vi "S4GUI_003.vi"(7 "Tab ObsEng":enum32{"Obs", "CCD modes", "Guider", "Eng"}(tab)) -> ()   [LabVIEW 2018] (continued)
                w2587 = enum16{"OFF", "ON"}."OFF" ("Frame Transfer")
                n1481 = property on="Frame Transfer" class="Enum (strict)"(error in=w2589, "DisabledEnum"=T12."Disabled and Grayed Out" ("Disabled"), "Value"=w2587) -> (error out=w2588:errorcluster)  [unwired: 1 in, 1 out]
              }
            }
            n1482 = property on="FT warning" class="Str"("Caption.Visible"=w2543) -> ()  [unwired: 2 in, 2 out]
            n1483 = call-dynamic "Write mode Adm.vi"("error in (no error)"=w2550, "mode Adm"=FALSE, "S4GUI in"=w2546) -> ("error out"=w2576:errorcluster, "S4GUI out"=w2578:refnum<class "S4GUI.lvclass">)  [unwired: 7 in]
            n1484 = local write "password 2"("" ("password")) -> ()
            n1485 = call-dynamic "Write SET request.vi"("error in (no error)"=w2576, "SET request"=FALSE, "S4GUI in"=w2578) -> ("error out"=w2575:errorcluster, "S4GUI out"=w2577:refnum<class "S4GUI.lvclass">)  [unwired: 7 in]
            n1486 = disable-structure shown="Disabled" {
              frame Disabled {
                n1487 = flat-sequence {
                  tunnel: _ -> [w2597]
                  tunnel: [w2597] -> _
                  frame #0 {
                    n1488 = local read "AQM"() -> (w2594:T4)
                    n1489 = Less Or Equal?(x=w2594, y=T4."NORMAL FAINT: Conventional; 1 MHz; Gain 2") -> (x <= y?=w2593:bool)
                    n1490 = Select(t=w2594, s=w2593, f=T4."SLOW BRIGHT: Conventional; 0.1 MHz; Gain 1" ("y")) -> (s? t:f=w2595:T4)
                    n1491 = local write "EM Gain"(u16 2 ("EM Gain")) -> ()
                    n1492 = local write "AQM"(w2595) -> ()
                  }
                }
              }
              frame Enabled {
              }
            }
            n1493 = flat-sequence {
              tunnel: w2575 -> [w2600]
              tunnel: [w2600] -> w2561
              tunnel: [w2599] -> w2558
              tunnel: [w2598] -> w2559
              frame #0 {
                w2598 = u16 2 ("EM Gain")
                w2599 = T4."NORMAL FAINT: Conventional; 1 MHz; Gain 2" ("AQM")
                n1494 = local write "EM Gain"(w2598) -> ()
                n1495 = local write "AQM"(w2599) -> ()
              }
            }
            n1496 = call-dynamic "Read CCD mode.vi"("error in (no error)"=w2561, "S4GUI in"=w2577) -> ("error out"=w2566:errorcluster, "CCD mode"=w2564:T30, "S4GUI out"=w2563:refnum<class "S4GUI.lvclass">)  [unwired: 7 in]
            n1497 = local read "SZM"() -> (w2560:T3)
            n1498 = Bundle By Name(cluster=w2564, "FTM"=w2544, "SZM"=w2560, "EM gain"=w2559, "AQM"=w2558) -> (w2565:T30)
            n1499 = call-dynamic "Write CCD mode.vi"("error in (no error)"=w2566, "CCD mode"=w2565, "S4GUI in"=w2563) -> ("error out"=w2568:errorcluster, "S4GUI out"=w2567:refnum<class "S4GUI.lvclass">)  [unwired: 7 in]
            n1500 = call-dynamic "LoadCCDmode.vi"("error in (no error)"=w2568, "S4GUI in"=w2567) -> ("error out"=w2570:errorcluster, "S4GUI out"=w2569:refnum<class "S4GUI.lvclass">)  [unwired: 8 in]
            n1501 = call-dynamic "Read Parameters CCD modes.vi"("error in (no error)"=w2570, "S4GUI in"=w2569) -> ("error out"=w2573:errorcluster, "Parameters CCD modes"=w2562:T5, "S4GUI out"=w2571:refnum<class "S4GUI.lvclass">)  [unwired: 7 in]
            n1502 = local write "Parameters CCD modes"(w2562) -> ()
            n1503 = call-dynamic "Read InfoCCDmode.vi"("error in (no error)"=w2573, "S4GUI in"=w2571) -> ("error out"=w2556:errorcluster, "InfoCCDmode"=w2572:T2, "S4GUI out"=w2557:refnum<class "S4GUI.lvclass">)  [unwired: 7 in]
            n1504 = local write "InfoCCDmode"(w2572) -> ()
            n1505 = call-dynamic "CalcTemp.vi"("error in (no error)"=w2556, "S4GUI in"=w2557) -> ("error out"=w2555:errorcluster, "S4GUI out"=w2553:refnum<class "S4GUI.lvclass">)  [unwired: 8 in]
            n1506 = call-dynamic "Read Prev Temp.vi"("error in (no error)"=w2555, "S4GUI in"=w2553) -> ("error out"=w2554:errorcluster, "Prev Temp"=w2551:dbl, "S4GUI out"=w2552:refnum<class "S4GUI.lvclass">)  [unwired: 7 in]
            n1507 = local write "Preview Temp."(w2551) -> ()
          }
          frame "Eng" {
            w2708 = T12."Disabled and Grayed Out" ("Disabled")
            # "Desabilita os botões SET."
            # "Entrou na aba  \"Eng\", ajusta para modo usuário normal..."
            n1508 = local write "password"("" ("password")) -> ()
            n1509 = call-dynamic "Write mode Adm.vi"("error in (no error)"=w2601, "mode Adm"=FALSE, "S4GUI in"=w2710) -> ("error out"=w2703:errorcluster, "S4GUI out"=w2706:refnum<class "S4GUI.lvclass">)  [unwired: 7 in]
            n1510 = property on="Set from Input ch1" class="Bool"("DisabledEnum"=w2708) -> ()  [unwired: 2 in, 2 out]
            n1511 = property on="Set from Input ch3" class="Bool"("DisabledEnum"=w2708) -> ()  [unwired: 2 in, 2 out]
            n1512 = property on="Set from Input ch2" class="Bool"("DisabledEnum"=w2708) -> ()  [unwired: 2 in, 2 out]
            n1513 = property on="Set from Input ch4" class="Bool"("DisabledEnum"=w2708) -> ()  [unwired: 2 in, 2 out]
            n1514 = local read "TARGET NAME WPSEL"() -> (w2659:enum16{"NONE", "OFF", "L/2", "L/4"})
            n1515 = call "Read Instrument.lvclass.vi"("error in (no error)"=w2703, "S4ACS_GUI in"=w2706) -> ("error out"=w2684:errorcluster, "Instrument.lvclass"=w2701:refnum<class "Instrument.lvclass">, "S4ACS_GUI out"=w2705:refnum<class "S4GUI.lvclass">)  [unwired: 7 in]
            n1516 = local read "TARGET NAME CALW"() -> (w2649:T9)
            n1517 = property on="TARGET NAME WPSEL" class="Enum (strict)"() -> ("RingText.Text"=w2657:string)  [unwired: 2 in, 2 out]
            n1518 = call "Read WPSEL.vi"("error in (no error)"=w2684, "Instrument in"=w2701) -> ("error out"=w2699:errorcluster, "Opt_Selector.lvclass"=w2697:refnum<class "Opt_Selector.lvclass">, "Instrument out"=w2700:refnum<class "Instrument.lvclass">)  [unwired: 7 in]
            n1519 = Build Array(-1.0 ("element"), 80.0 ("element"), 0.0 ("element"), 160.0 ("element")) -> (w2660:dbl[])
            n1520 = property on="TARGET NAME CALW" class="Enum (strict)"() -> ("RingText.Text"=w2648:string)  [unwired: 2 in, 2 out]
            n1521 = Build Array(-1.0 ("element"), 0.0 ("element"), 72.0 ("element"), 144.0 ("element"), 216.0 ("element"), 288.0 ("element")) -> (w2652:dbl[])
            n1522 = Index Array "Index Array"(array=w2660, index=w2659) -> (element=w2658:dbl)
            n1523 = call "Write target name.vi"("error in (no error)"=w2699, "target name"=w2657, "Optics in"=w2697) -> ("error out"=w2698:errorcluster, "Optics out"=w2696:refnum<class "Opt_Selector.lvclass">)  [unwired: 7 in]
            n1524 = Index Array(array=w2652, index=w2649) -> (element=w2647:dbl)
            n1525 = call "Write target.vi"("error in (no error)"=w2698, "target"=w2658, "Optics in"=w2696) -> ("error out"=w2694:errorcluster, "Optics out"=w2695:refnum<class "Opt_Selector.lvclass">)  [unwired: 7 in]
            n1526 = call "Write WPSEL.vi"("error in (no error)"=w2694, "Opt_Selector.lvclass"=w2695, "Instrument in"=w2700) -> ("error out"=w2693:errorcluster, "Instrument out"=w2692:refnum<class "Instrument.lvclass">)  [unwired: 7 in]
            n1527 = call "Read CALW.vi"("error in (no error)"=w2693, "Instrument in"=w2692) -> ("error out"=w2690:errorcluster, "Opt_Selector.lvclass"=w2688:refnum<class "Opt_Selector.lvclass">, "Instrument out"=w2685:refnum<class "Instrument.lvclass">)  [unwired: 7 in]
            n1528 = call "Write target name.vi"("error in (no error)"=w2690, "target name"=w2648, "Optics in"=w2688) -> ("error out"=w2691:errorcluster, "Optics out"=w2687:refnum<class "Opt_Selector.lvclass">)  [unwired: 7 in]
            n1529 = call "Write target.vi"("error in (no error)"=w2691, "target"=w2647, "Optics in"=w2687) -> ("error out"=w2689:errorcluster, "Optics out"=w2686:refnum<class "Opt_Selector.lvclass">)  [unwired: 7 in]
            n1530 = local read "TARGET NAME ASEL"() -> (w2641:enum16{"NONE", "OFF", "ON"})
            n1531 = call "Write CALW.vi"("error in (no error)"=w2689, "Opt_Selector.lvclass"=w2686, "Instrument in"=w2685) -> ("error out"=w2681:errorcluster, "Instrument out"=w2682:refnum<class "Instrument.lvclass">)  [unwired: 7 in]
            n1532 = property on="TARGET NAME ASEL" class="Enum (strict)"() -> ("RingText.Text"=w2642:string)  [unwired: 2 in, 2 out]
            n1533 = Build Array(-1.0 ("element"), 0.0 ("element"), 30.0 ("element")) -> (w2643:dbl[])
            n1534 = Index Array(array=w2643, index=w2641) -> (element=w2640:dbl)
            n1535 = call "Read ASEL.vi"("error in (no error)"=w2681, "Instrument in"=w2682) -> ("error out"=w2680:errorcluster, "Opt_Selector.lvclass"=w2678:refnum<class "Opt_Selector.lvclass">, "Instrument out"=w2675:refnum<class "Instrument.lvclass">)  [unwired: 7 in]
            n1536 = call "Write target name.vi"("error in (no error)"=w2680, "target name"=w2642, "Optics in"=w2678) -> ("error out"=w2683:errorcluster, "Optics out"=w2677:refnum<class "Opt_Selector.lvclass">)  [unwired: 7 in]
            n1537 = call "Write target.vi"("error in (no error)"=w2683, "target"=w2640, "Optics in"=w2677) -> ("error out"=w2679:errorcluster, "Optics out"=w2676:refnum<class "Opt_Selector.lvclass">)  [unwired: 7 in]
            n1538 = call "Write ASEL.vi"("error in (no error)"=w2679, "Opt_Selector.lvclass"=w2676, "Instrument in"=w2675) -> ("error out"=w2674:errorcluster, "Instrument out"=w2673:refnum<class "Instrument.lvclass">)  [unwired: 7 in]
            n1539 = local read "GMIR_target"() -> (w2634:dbl)
            n1540 = local read "GFOC_target"() -> (w2635:dbl)
            n1541 = call "Read GFOC.vi"("error in (no error)"=w2674, "Instrument in"=w2673) -> ("error out"=w2638:errorcluster, "Opt_Continuous.lvclass"=w2639:refnum<class "Opt_Continuous.lvclass">, "Instrument out"=w2670:refnum<class "Instrument.lvclass">)  [unwired: 7 in]
            n1542 = call "Write target.vi"("error in (no error)"=w2638, "target"=w2635, "Optics in"=w2639) -> ("error out"=w2672:errorcluster, "Optics out"=w2669:refnum<class "Opt_Continuous.lvclass">)  [unwired: 7 in]
            n1543 = call "Write GFOC.vi"("error in (no error)"=w2672, "Opt_Continuous.lvclass"=w2669, "Instrument in"=w2670) -> ("error out"=w2671:errorcluster, "Instrument out"=w2668:refnum<class "Instrument.lvclass">)  [unwired: 7 in]
            n1544 = call "Read GMIR.vi"("error in (no error)"=w2671, "Instrument in"=w2668) -> ("error out"=w2636:errorcluster, "Opt_Continuous.lvclass"=w2637:refnum<class "Opt_Continuous.lvclass">, "Instrument out"=w2667:refnum<class "Instrument.lvclass">)  [unwired: 7 in]
            n1545 = call "Write target.vi"("error in (no error)"=w2636, "target"=w2634, "Optics in"=w2637) -> ("error out"=w2665:errorcluster, "Optics out"=w2666:refnum<class "Opt_Continuous.lvclass">)  [unwired: 7 in]
            n1546 = local read "TARGET NAME WPROT"() -> (w2603:T10)
            n1547 = call "Write GMIR.vi"("error in (no error)"=w2665, "Opt_Continuous.lvclass"=w2666, "Instrument in"=w2667) -> ("error out"=w2630:errorcluster, "Instrument out"=w2629:refnum<class "Instrument.lvclass">)  [unwired: 7 in]
            n1548 = property on="TARGET NAME WPROT" class="Enum (strict)"() -> ("RingText.Text"=w2602:string)  [unwired: 2 in, 2 out]
            n1549 = call "Read WPROT.vi"("error in (no error)"=w2630, "Instrument in"=w2629) -> ("error out"=w2627:errorcluster, "Opt_Selector.lvclass"=w2631:refnum<class "Opt_Selector.lvclass">, "Instrument out"=w2628:refnum<class "Instrument.lvclass">)  [unwired: 7 in]
            n1550 = Build Array(-1.0 ("element"), 0.0 ("element"), 22.5 ("element"), 45.0 ("element"), 67.5 ("element"), 90.0 ("element"), 112.5 ("element"), 135.0 ("element"), 157.5 ("element"), 180.0 ("element"), 202.5 ("element"), 225.0 ("element"), 247.5 ("element"), 270.0 ("element"), 292.5 ("element"), 315.0 ("element"), 337.5 ("element")) -> (w2616:dbl[])
            n1551 = Index Array(array=w2616, index=w2603) -> (element=w2604:dbl)
            n1552 = call "Write target name.vi"("error in (no error)"=w2627, "target name"=w2602, "Optics in"=w2631) -> ("error out"=w2626:errorcluster, "Optics out"=w2633:refnum<class "Opt_Selector.lvclass">)  [unwired: 7 in]
            n1553 = call "Write target.vi"("error in (no error)"=w2626, "target"=w2604, "Optics in"=w2633) -> ("error out"=w2625:errorcluster, "Optics out"=w2632:refnum<class "Opt_Selector.lvclass">)  [unwired: 7 in]
            n1554 = call "Write WPROT.vi"("error in (no error)"=w2625, "Opt_Selector.lvclass"=w2632, "Instrument in"=w2628) -> ("error out"=w2623:errorcluster, "Instrument out"=w2624:refnum<class "Instrument.lvclass">)  [unwired: 7 in]
            n1555 = call "Write Instrument.lvclass.vi"("error in (no error)"=w2623, "Instrument.lvclass"=w2624, "S4ACS_GUI in"=w2705) -> ("error out"=w2702:errorcluster, "S4ACS_GUI out"=w2704:refnum<class "S4GUI.lvclass">)  [unwired: 7 in]
          }
          frame Default {
            n1556 = call "Read Instrument.lvclass.vi"("error in (no error)"=w2714, "S4ACS_GUI in"=w2719) -> ("error out"=w2713:errorcluster, "Instrument.lvclass"=w2718:refnum<class "Instrument.lvclass">, "S4ACS_GUI out"=w2715:refnum<class "S4GUI.lvclass">)  [unwired: 7 in]
            n1557 = call "Read WPSEL.vi"("Instrument in"=w2718) -> ("Opt_Selector.lvclass"=w2717:refnum<class "Opt_Selector.lvclass">)  [unwired: 8 in, 2 out]
            n1558 = call "Read name_pos.vi"("Optics in"=w2717) -> ("name_pos"=w2716:string)  [unwired: 8 in, 2 out]
            n1559 = case shown="\"OFF\", Default" w2716 {
              tunnel: [w2721 w2723 w2725] -> w2712
              tunnel: ["Lambda/4" ("Ring Text.Text") "Lambda/2" ("Ring Text.Text") "OFF" ("Ring Text.Text")] -> w2711
              frame "L/4" {
                w2721 = u16 2 items=["OFF", "Lambda/2", "Lambda/4"] ("Lambda Selector")
              }
              frame "L/2" {
                w2723 = u16 1 items=["OFF", "Lambda/2", "Lambda/4"] ("Lambda Selector")
              }
              frame "OFF", Default {
                w2725 = u16 0 items=["OFF", "Lambda/2", "Lambda/4"] ("Lambda Selector")
              }
            }
            n1560 = property on="Lambda Selector" class="Ring (strict)"("Value"=w2712, "RingText.Text"=w2711) -> ()  [unwired: 2 in, 2 out]
          }
        }
      }
      event "S4ICS protocol": Value Change {
        # "2024-04-04: Não se usa mais o ID para configurar a comunicação..."
        # "TCP-IP"
        # "ZeroMQ"
        # "Inicializar nova comunicação, de acordo\n com valor de S4ICS mode\n\nServer.Write id (T=13 ou F=5)\nInstrument.Init"
        # "Parar a comunciação atual\nServer.End"
        n1561 = event-data() -> ("NewVal"=w2728:bool)  [unwired: 1 in, 5 out]
        n1562 = call "Read Instrument.lvclass.vi"("error in (no error)"=w2738, "S4ACS_GUI in"=w2739) -> ("error out"=w2733:errorcluster, "Instrument.lvclass"=w2736:refnum<class "Instrument.lvclass">, "S4ACS_GUI out"=w2737:refnum<class "S4GUI.lvclass">)  [unwired: 7 in]
        n1563 = call-dynamic "End.vi"("error in (no error)"=w2733, "Server in"=w2736) -> ("error out"=w2732:errorcluster, "Server out"=w2735:refnum<class "Instrument.lvclass">)  [unwired: 8 in]
        n1564 = Select(t=u32 13, s=w2728, f=u32 5) -> (s? t:f=w2742:u32)
        n1565 = call-dynamic "Write id.vi"("error in (no error)"=w2732, "id"=w2742, "Server in"=w2735) -> ("error out"=w2731:errorcluster, "Server out"=w2734:refnum<class "Instrument.lvclass">)  [unwired: 7 in]
        n1566 = call-dynamic "Initialize.vi"("error in (no error)"=w2731, "Instrument in"=w2734) -> ("error out"=w2729:errorcluster, "Instrument out"=w2730:refnum<class "Instrument.lvclass">)  [unwired: 8 in]
        n1567 = call "Write Instrument.lvclass.vi"("error in (no error)"=w2729, "Instrument.lvclass"=w2730, "S4ACS_GUI in"=w2737) -> ("error out"=w2726:errorcluster, "S4ACS_GUI out"=w2727:refnum<class "S4GUI.lvclass">)  [unwired: 7 in]
      }
      event "Set from Input ch1": Value Change {
        # "ACS"
        # "GUI"
        # "EM_MODE = E.M."
        # "Readou Rate:\n30         0\n20         1     \n10         2\n1           3"
        # "EM_MODE = Conv"
        # "Readou Rate:\n1         0\n0.1      1"
        # "Readou Rate:\n1         0\n0.1      1     \n10       2\n20       3\n30       4"
        n1568 = event-data() -> ()  [unwired: 1 in, 6 out]
        n1569 = local read "Input Cluster"() -> (w2767:T8)
        n1570 = Unbundle By Name(w2767) -> ("Parameters"=w2766:T5)
        n1571 = Unbundle By Name(w2766) -> ("Image \nInitial Line"=w2794:u16, "Image\nInitial Column"=w2793:u16, "Image\nFinal Line"=w2792:u16, "Image\nFInal Column"=w2791:u16, "Vertical\nBinning"=w2790:u16, "Horizontal\nBinning"=w2789:u16, "Pre-amplification\nGain"=w2788:u8, "CCD\nEM Gain"=w2787:u16, "Readout\nRate"=w2786:u8, "Shutter\nOpenning Time"=w2785:i32, "Shutter\nClosing Time"=w2784:i32, "Vertical\nShift Speed"=w2783:u8, "Read\nMode"=w2782:u8, "Vertical\nClock Voltage"=w2781:u8, "A/D \nChannel"=w2780:u32, "Shutter\nMode"=w2779:u16, "Shutter\nTTL"=w2778:u16, "Trigger\nMode"=w2777:u16, "Frame\nTransfer"=w2758:bool, "Acquisition\nMode"=w2776:u8, "CCD \nEM Mode"=w2775:u8)
        n1572 = call-dynamic "Write User Event.vi"("error in (no error)"=w2746, "User Event"="SET CCD CONFIG CHANNEL1 ", "S4GUI in"=w2747) -> ("error out"=w2744:errorcluster, "S4GUI out"=w2745:refnum<class "S4GUI.lvclass">)  [unwired: 7 in]
        n1573 = call-dynamic "Read AcquisitionA.vi"("error in (no error)"=w2744, "S4ACS_GUI in"=w2745) -> ("error out"=w2810:errorcluster, "Acquisition.lvclass"=w2813:refnum<class "Acquisition.lvclass">, "S4ACS_GUI out"=w2814:refnum<class "S4GUI.lvclass">)  [unwired: 7 in]
        n1574 = call-dynamic "Read Channel.vi"("error in (no error)"=w2810, "Acquisition in"=w2813) -> ("error out"=w2809:errorcluster, "Channel.lvclass"=w2811:refnum<class "Channel.lvclass">, "Acquisition out"=w2812:refnum<class "Acquisition.lvclass">)  [unwired: 7 in]
        n1575 = call-dynamic "Read Interface.vi"("error in (no error)"=w2809, "Channel in"=w2811) -> ("error out"=w2757:errorcluster, "Interface.lvclass"=w2759:refnum<class "Interface.lvclass">, "Channel out"=w2754:refnum<class "Channel.lvclass">)  [unwired: 7 in]
        n1576 = call-dynamic "Write PREV_FT.vi"("error in (no error)"=w2757, "PREV_FT"=w2758, "Interface in"=w2759) -> ("error out"=w2756:errorcluster, "Interface out"=w2755:refnum<class "Interface.lvclass">)  [unwired: 7 in]
        n1577 = call-dynamic "Read target cluster.vi"("error in (no error)"=w2756, "Channel in"=w2754) -> ("error out"=w2752:errorcluster, "target cluster"=w2750:T31, "Channel out"=w2751:refnum<class "Channel.lvclass">)  [unwired: 7 in]
        n1578 = Bundle By Name(cluster=w2750, "INITIAL_LINE"=w2794, "INITIAL_COLUMN"=w2793, "FINAL_LINE"=w2792, "FINAL_COLUMN"=w2791, "VBIN"=w2790, "HBIN"=w2789, "PREAMP"=w2788, "EM_GAIN"=w2787, "READOUT_RATE"=w2786, "SHUTTER_OPENING_TIME"=w2785, "SHUTTER_CLOSING_TIME"=w2784, "VERTICAL_SHIFT_SPEED"=w2783, "READ_MODE"=w2782, "VERTICAL_CLOCK_VOLTAGE"=w2781, "AD_CHANNEL"=w2780, "SHUTTER_MODE"=w2779, "SHUTTER_TTL"=w2778, "TRIGGER_MODE"=w2777, "FRAME_TRANSFER"=w2758, "ACQUISITION_MODE"=w2776, "EM_MODE"=w2775) -> (w2749:T31)
        n1579 = call-dynamic "Write target cluster.vi"("error in (no error)"=w2752, "target cluster"=w2749, "Channel in"=w2751) -> ("error out"=w2748:errorcluster, "Channel out"=w2753:refnum<class "Channel.lvclass">)  [unwired: 7 in]
        n1580 = Flatten To String(anything=w2749, error in (no error)=w2748) -> (data string=w2798:string, error out=w2797:errorcluster)  [unwired: 2 in, 1 out]
        n1581 = call "Write flatted cluster.vi"("error in (no error)"=w2797, "flatted cluster"=w2798, "Interface in"=w2755) -> ("error out"=w2796:errorcluster, "Interface out"=w2795:refnum<class "Interface.lvclass">)  [unwired: 7 in]
        n1582 = call-dynamic "Write Interface.vi"("error in (no error)"=w2796, "Interface.lvclass"=w2795, "Channel in"=w2753) -> ("error out"=w2770:errorcluster, "Channel out"=w2773:refnum<class "Channel.lvclass">)  [unwired: 7 in]
        n1583 = call "Write section_name.vi"("error in (no error)"=w2770, "section_name"="CCD_ACS1", "Channel in"=w2773) -> ("error out"=w2769:errorcluster, "Channel out"=w2772:refnum<class "Channel.lvclass">)  [unwired: 7 in]
        n1584 = call-dynamic "save config.vi"("error in (no error)"=w2769, "file config"="lastsaved.cfg", "Channel in"=w2772) -> ("error out"=w2768:errorcluster, "Channel out"=w2771:refnum<class "Channel.lvclass">)  [unwired: 7 in]
        n1585 = call-dynamic "Read State Machine.vi"("error in (no error)"=w2768, "Device in"=w2771) -> ("error out"=w2805:errorcluster, "State Machine.lvclass"=w2807:refnum<class "State Machine.lvclass">, "Device out"=w2808:refnum<class "Channel.lvclass">)  [unwired: 7 in]
        n1586 = call-dynamic "Write State.vi"("error in (no error)"=w2805, "State"=60, "State Machine in"=w2807) -> ("error out"=w2804:errorcluster, "State Machine out"=w2806:refnum<class "State Machine.lvclass">)  [unwired: 7 in]
        n1587 = call-dynamic "Write State Machine.vi"("error in (no error)"=w2804, "State Machine.lvclass"=w2806, "Device in"=w2808) -> ("error out"=w2801:errorcluster, "Device out"=w2802:refnum<class "Channel.lvclass">)  [unwired: 7 in]
        n1588 = call-dynamic "Write Channel.vi"("error in (no error)"=w2801, "Channel.lvclass"=w2802, "Acquisition in"=w2812) -> ("error out"=w2800:errorcluster, "Acquisition out"=w2799:refnum<class "Acquisition.lvclass">)  [unwired: 7 in]
        n1589 = call-dynamic "Write AcquisitionA.vi"("error in (no error)"=w2800, "Acquisition.lvclass"=w2799, "S4ACS_GUI in"=w2814) -> ("error out"=w2761:errorcluster, "S4ACS_GUI out"=w2762:refnum<class "S4GUI.lvclass">)  [unwired: 7 in]
        n1590 = call "Write cfg file.vi"("error in (no error)"=w2761, "cfg file"="lastsaved.cfg", "S4ACS_GUI in"=w2762) -> ("error out"=w2764:errorcluster, "S4ACS_GUI out"=w2765:refnum<class "S4GUI.lvclass">)  [unwired: 7 in]
      }
      event "Input Cluster.Parameters.CCD \nEM Mode": Value Change {
        n1591 = event-data() -> ()  [unwired: 1 in, 6 out]
        n1592 = local read "Input Cluster"() -> (w2829:T8)
        n1593 = Unbundle By Name(w2829) -> ("Parameters"=w2830:T5)
        n1594 = Unbundle By Name(w2830) -> ("Readout\nRate"=→"Readout\nRate":u8, "CCD \nEM Mode"=w2824:u8)
        n1595 = case shown="0, Default" w2824 {
          tunnel: [string[] ["30 MHz", "20 MHz", "10 MHz", "1 MHz"] ("Strings []") string[] ["1 MHz", "0.1 MHz"] ("Strings []")] -> w2823
          tunnel: [u8 3 u8 0] -> w2822
          frame 0, Default {
          }
          frame 1 {
          }
        }
        n1596 = local read "Cameras Cluster"() -> (w2817:T7)
        n1597 = flat-sequence {
          tunnel: w2822 -> [w2832]
          tunnel: w2823 -> [w2831]
          tunnel: w2824 -> [w2833]
          tunnel: [w2833] -> w2821
          tunnel: [w2832] -> w2819
          tunnel: w2830 -> [w2839]
          tunnel: [w2838] -> w2828
          tunnel: w2821 -> [w2834]
          tunnel: w2819 -> [w2835]
          tunnel: w2818 -> [w2837]
          tunnel: [w2836] -> w2816
          frame #0 {
            n1598 = property on="Readout\nRate" class="Ring (strict)"("Strings []"=w2831) -> ()  [unwired: 2 in, 2 out]
            n1599 = property on="Readout Rate" class="Ring (strict)"("Strings []"=w2831) -> ()  [unwired: 2 in, 2 out]
            n1600 = property on="Readout Rate 4" class="Ring (strict)"("Strings []"=w2831) -> ()  [unwired: 2 in, 2 out]
            n1601 = property on="Readout Rate 2" class="Ring (strict)"("Strings []"=w2831) -> ()  [unwired: 2 in, 2 out]
            n1602 = property on="Readout Rate 3" class="Ring (strict)"("Strings []"=w2831) -> ()  [unwired: 2 in, 2 out]
          }
          frame #1 {
            n1603 = Bundle By Name(cluster=w2837, "Readout Rate"=w2835, "Read Mode"=w2834) -> (w2836:T32)
            n1604 = Bundle By Name(cluster=w2839, "Readout\nRate"=w2835, "CCD \nEM Mode"=w2834) -> (w2838:T5)
          }
        }
        n1605 = Unbundle By Name(w2817) -> ("Current Configuration"=w2818:T32)
        n1606 = Bundle By Name(cluster=w2829, "Parameters"=w2828) -> (w2827:T8)
        n1607 = local write "Input Cluster"(w2827) -> ()
        n1608 = Bundle By Name(cluster=w2817, "Current Configuration"=w2816) -> (w2815:T7)
        n1609 = local write "Cameras Cluster"(w2815) -> ()
      }
      event "Set from Input ch2": Value Change {
        n1610 = event-data() -> ()  [unwired: 1 in, 6 out]
        n1611 = local read "Input Cluster"() -> (w2868:T8)
        n1612 = Unbundle By Name(w2868) -> ("Parameters"=w2867:T5)
        n1613 = call-dynamic "Write User Event.vi"("error in (no error)"=w2846, "User Event"="SET CCD CONFIG CHANNEL2 ", "S4GUI in"=w2847) -> ("error out"=w2844:errorcluster, "S4GUI out"=w2845:refnum<class "S4GUI.lvclass">)  [unwired: 7 in]
        n1614 = Unbundle By Name(w2867) -> ("Image \nInitial Line"=w2895:u16, "Image\nInitial Column"=w2894:u16, "Image\nFinal Line"=w2893:u16, "Image\nFInal Column"=w2892:u16, "Vertical\nBinning"=w2891:u16, "Horizontal\nBinning"=w2890:u16, "Pre-amplification\nGain"=w2889:u8, "CCD\nEM Gain"=w2888:u16, "Readout\nRate"=w2887:u8, "Shutter\nOpenning Time"=w2886:i32, "Shutter\nClosing Time"=w2885:i32, "Vertical\nShift Speed"=w2884:u8, "Read\nMode"=w2883:u8, "Vertical\nClock Voltage"=w2882:u8, "A/D \nChannel"=w2881:u32, "Shutter\nMode"=w2880:u16, "Shutter\nTTL"=w2879:u16, "Trigger\nMode"=w2878:u16, "Frame\nTransfer"=w2858:bool, "Acquisition\nMode"=w2877:u8, "CCD \nEM Mode"=w2876:u8)
        n1615 = call "Read AcquisitionB.vi"("error in (no error)"=w2844, "S4ACS_GUI in"=w2845) -> ("error out"=w2911:errorcluster, "Acquisition.lvclass"=w2914:refnum<class "Acquisition.lvclass">, "S4ACS_GUI out"=w2915:refnum<class "S4GUI.lvclass">)  [unwired: 7 in]
        n1616 = call-dynamic "Read Channel.vi"("error in (no error)"=w2911, "Acquisition in"=w2914) -> ("error out"=w2910:errorcluster, "Channel.lvclass"=w2912:refnum<class "Channel.lvclass">, "Acquisition out"=w2913:refnum<class "Acquisition.lvclass">)  [unwired: 7 in]
        n1617 = call-dynamic "Read Interface.vi"("error in (no error)"=w2910, "Channel in"=w2912) -> ("error out"=w2859:errorcluster, "Interface.lvclass"=w2860:refnum<class "Interface.lvclass">, "Channel out"=w2855:refnum<class "Channel.lvclass">)  [unwired: 7 in]
        n1618 = call-dynamic "Write PREV_FT.vi"("error in (no error)"=w2859, "PREV_FT"=w2858, "Interface in"=w2860) -> ("error out"=w2852:errorcluster, "Interface out"=w2850:refnum<class "Interface.lvclass">)  [unwired: 7 in]
        n1619 = call-dynamic "Read target cluster.vi"("error in (no error)"=w2852, "Channel in"=w2855) -> ("error out"=w2857:errorcluster, "target cluster"=w2854:T31, "Channel out"=w2856:refnum<class "Channel.lvclass">)  [unwired: 7 in]
        n1620 = Bundle By Name(cluster=w2854, "INITIAL_LINE"=w2895, "INITIAL_COLUMN"=w2894, "FINAL_LINE"=w2893, "FINAL_COLUMN"=w2892, "VBIN"=w2891, "HBIN"=w2890, "PREAMP"=w2889, "EM_GAIN"=w2888, "READOUT_RATE"=w2887, "SHUTTER_OPENING_TIME"=w2886, "SHUTTER_CLOSING_TIME"=w2885, "VERTICAL_SHIFT_SPEED"=w2884, "READ_MODE"=w2883, "VERTICAL_CLOCK_VOLTAGE"=w2882, "AD_CHANNEL"=w2881, "SHUTTER_MODE"=w2880, "SHUTTER_TTL"=w2879, "TRIGGER_MODE"=w2878, "FRAME_TRANSFER"=w2858, "ACQUISITION_MODE"=w2877, "EM_MODE"=w2876) -> (w2853:T31)
        n1621 = call-dynamic "Write target cluster.vi"("error in (no error)"=w2857, "target cluster"=w2853, "Channel in"=w2856) -> ("error out"=w2851:errorcluster, "Channel out"=w2849:refnum<class "Channel.lvclass">)  [unwired: 7 in]
        n1622 = Flatten To String(anything=w2853, error in (no error)=w2851) -> (data string=w2899:string, error out=w2898:errorcluster)  [unwired: 2 in, 1 out]
        n1623 = call "Write flatted cluster.vi"("error in (no error)"=w2898, "flatted cluster"=w2899, "Interface in"=w2850) -> ("error out"=w2897:errorcluster, "Interface out"=w2896:refnum<class "Interface.lvclass">)  [unwired: 7 in]
        n1624 = call-dynamic "Write Interface.vi"("error in (no error)"=w2897, "Interface.lvclass"=w2896, "Channel in"=w2849) -> ("error out"=w2871:errorcluster, "Channel out"=w2874:refnum<class "Channel.lvclass">)  [unwired: 7 in]
        n1625 = call "Write section_name.vi"("error in (no error)"=w2871, "section_name"="CCD_ACS2", "Channel in"=w2874) -> ("error out"=w2870:errorcluster, "Channel out"=w2873:refnum<class "Channel.lvclass">)  [unwired: 7 in]
        n1626 = call-dynamic "save config.vi"("error in (no error)"=w2870, "file config"="lastsaved.cfg", "Channel in"=w2873) -> ("error out"=w2869:errorcluster, "Channel out"=w2872:refnum<class "Channel.lvclass">)  [unwired: 7 in]
        n1627 = call-dynamic "Read State Machine.vi"("error in (no error)"=w2869, "Device in"=w2872) -> ("error out"=w2906:errorcluster, "State Machine.lvclass"=w2908:refnum<class "State Machine.lvclass">, "Device out"=w2909:refnum<class "Channel.lvclass">)  [unwired: 7 in]
        n1628 = call-dynamic "Write State.vi"("error in (no error)"=w2906, "State"=60, "State Machine in"=w2908) -> ("error out"=w2905:errorcluster, "State Machine out"=w2907:refnum<class "State Machine.lvclass">)  [unwired: 7 in]
        n1629 = call-dynamic "Write State Machine.vi"("error in (no error)"=w2905, "State Machine.lvclass"=w2907, "Device in"=w2909) -> ("error out"=w2902:errorcluster, "Device out"=w2903:refnum<class "Channel.lvclass">)  [unwired: 7 in]
        n1630 = call-dynamic "Write Channel.vi"("error in (no error)"=w2902, "Channel.lvclass"=w2903, "Acquisition in"=w2913) -> ("error out"=w2901:errorcluster, "Acquisition out"=w2900:refnum<class "Acquisition.lvclass">)  [unwired: 7 in]
        n1631 = call "Write AcquisitionB.vi"("error in (no error)"=w2901, "Acquisition.lvclass"=w2900, "S4ACS_GUI in"=w2915) -> ("error out"=w2861:errorcluster, "S4ACS_GUI out"=w2862:refnum<class "S4GUI.lvclass">)  [unwired: 7 in]
        n1632 = call "Write cfg file.vi"("error in (no error)"=w2861, "cfg file"="lastsaved.cfg", "S4ACS_GUI in"=w2862) -> ("error out"=w2864:errorcluster, "S4ACS_GUI out"=w2865:refnum<class "S4GUI.lvclass">)  [unwired: 7 in]
      }
      event "Set from Input ch3": Value Change {
        n1633 = event-data() -> ()  [unwired: 1 in, 6 out]
        n1634 = local read "Input Cluster"() -> (w2940:T8)
        n1635 = Unbundle By Name(w2940) -> ("Parameters"=w2939:T5)
        n1636 = call-dynamic "Write User Event.vi"("error in (no error)"=w2918, "User Event"="SET CCD CONFIG CHANNEL 3 ", "S4GUI in"=w2919) -> ("error out"=w2916:errorcluster, "S4GUI out"=w2917:refnum<class "S4GUI.lvclass">)  [unwired: 7 in]
        n1637 = Unbundle By Name(w2939) -> ("Image \nInitial Line"=w2967:u16, "Image\nInitial Column"=w2966:u16, "Image\nFinal Line"=w2965:u16, "Image\nFInal Column"=w2964:u16, "Vertical\nBinning"=w2963:u16, "Horizontal\nBinning"=w2962:u16, "Pre-amplification\nGain"=w2961:u8, "CCD\nEM Gain"=w2960:u16, "Readout\nRate"=w2959:u8, "Shutter\nOpenning Time"=w2958:i32, "Shutter\nClosing Time"=w2957:i32, "Vertical\nShift Speed"=w2956:u8, "Read\nMode"=w2955:u8, "Vertical\nClock Voltage"=w2954:u8, "A/D \nChannel"=w2953:u32, "Shutter\nMode"=w2952:u16, "Shutter\nTTL"=w2951:u16, "Trigger\nMode"=w2950:u16, "Frame\nTransfer"=w2930:bool, "Acquisition\nMode"=w2949:u8, "CCD \nEM Mode"=w2948:u8)
        n1638 = call-dynamic "Read AcquisitionC.vi"("error in (no error)"=w2916, "S4ACS_GUI in"=w2917) -> ("error out"=w2983:errorcluster, "Acquisition.lvclass"=w2986:refnum<class "Acquisition.lvclass">, "S4ACS_GUI out"=w2987:refnum<class "S4GUI.lvclass">)  [unwired: 7 in]
        n1639 = call-dynamic "Read Channel.vi"("error in (no error)"=w2983, "Acquisition in"=w2986) -> ("error out"=w2982:errorcluster, "Channel.lvclass"=w2984:refnum<class "Channel.lvclass">, "Acquisition out"=w2985:refnum<class "Acquisition.lvclass">)  [unwired: 7 in]
        n1640 = call-dynamic "Read Interface.vi"("error in (no error)"=w2982, "Channel in"=w2984) -> ("error out"=w2931:errorcluster, "Interface.lvclass"=w2932:refnum<class "Interface.lvclass">, "Channel out"=w2927:refnum<class "Channel.lvclass">)  [unwired: 7 in]
        n1641 = call-dynamic "Write PREV_FT.vi"("error in (no error)"=w2931, "PREV_FT"=w2930, "Interface in"=w2932) -> ("error out"=w2921:errorcluster, "Interface out"=w2928:refnum<class "Interface.lvclass">)  [unwired: 7 in]
        n1642 = call-dynamic "Read target cluster.vi"("error in (no error)"=w2921, "Channel in"=w2927) -> ("error out"=w2929:errorcluster, "target cluster"=w2923:T31, "Channel out"=w2926:refnum<class "Channel.lvclass">)  [unwired: 7 in]
        n1643 = Bundle By Name(cluster=w2923, "INITIAL_LINE"=w2967, "INITIAL_COLUMN"=w2966, "FINAL_LINE"=w2965, "FINAL_COLUMN"=w2964, "VBIN"=w2963, "HBIN"=w2962, "PREAMP"=w2961, "EM_GAIN"=w2960, "READOUT_RATE"=w2959, "SHUTTER_OPENING_TIME"=w2958, "SHUTTER_CLOSING_TIME"=w2957, "VERTICAL_SHIFT_SPEED"=w2956, "READ_MODE"=w2955, "VERTICAL_CLOCK_VOLTAGE"=w2954, "AD_CHANNEL"=w2953, "SHUTTER_MODE"=w2952, "SHUTTER_TTL"=w2951, "TRIGGER_MODE"=w2950, "FRAME_TRANSFER"=w2930, "ACQUISITION_MODE"=w2949, "EM_MODE"=w2948) -> (w2922:T31)
        n1644 = call-dynamic "Write target cluster.vi"("error in (no error)"=w2929, "target cluster"=w2922, "Channel in"=w2926) -> ("error out"=w2924:errorcluster, "Channel out"=w2925:refnum<class "Channel.lvclass">)  [unwired: 7 in]
        n1645 = Flatten To String(anything=w2922, error in (no error)=w2924) -> (data string=w2971:string, error out=w2970:errorcluster)  [unwired: 2 in, 1 out]
        n1646 = call "Write flatted cluster.vi"("error in (no error)"=w2970, "flatted cluster"=w2971, "Interface in"=w2928) -> ("error out"=w2969:errorcluster, "Interface out"=w2968:refnum<class "Interface.lvclass">)  [unwired: 7 in]
        n1647 = call-dynamic "Write Interface.vi"("error in (no error)"=w2969, "Interface.lvclass"=w2968, "Channel in"=w2925) -> ("error out"=w2943:errorcluster, "Channel out"=w2946:refnum<class "Channel.lvclass">)  [unwired: 7 in]
        n1648 = call "Write section_name.vi"("error in (no error)"=w2943, "section_name"="CCD_ACS3", "Channel in"=w2946) -> ("error out"=w2942:errorcluster, "Channel out"=w2945:refnum<class "Channel.lvclass">)  [unwired: 7 in]
        n1649 = call-dynamic "save config.vi"("error in (no error)"=w2942, "file config"="lastsaved.cfg", "Channel in"=w2945) -> ("error out"=w2941:errorcluster, "Channel out"=w2944:refnum<class "Channel.lvclass">)  [unwired: 7 in]
        n1650 = call-dynamic "Read State Machine.vi"("error in (no error)"=w2941, "Device in"=w2944) -> ("error out"=w2978:errorcluster, "State Machine.lvclass"=w2980:refnum<class "State Machine.lvclass">, "Device out"=w2981:refnum<class "Channel.lvclass">)  [unwired: 7 in]
        n1651 = call-dynamic "Write State.vi"("error in (no error)"=w2978, "State"=60, "State Machine in"=w2980) -> ("error out"=w2977:errorcluster, "State Machine out"=w2979:refnum<class "State Machine.lvclass">)  [unwired: 7 in]
        n1652 = call-dynamic "Write State Machine.vi"("error in (no error)"=w2977, "State Machine.lvclass"=w2979, "Device in"=w2981) -> ("error out"=w2974:errorcluster, "Device out"=w2975:refnum<class "Channel.lvclass">)  [unwired: 7 in]
        n1653 = call-dynamic "Write Channel.vi"("error in (no error)"=w2974, "Channel.lvclass"=w2975, "Acquisition in"=w2985) -> ("error out"=w2973:errorcluster, "Acquisition out"=w2972:refnum<class "Acquisition.lvclass">)  [unwired: 7 in]
        n1654 = call-dynamic "Write AcquisitionC.vi"("error in (no error)"=w2973, "Acquisition.lvclass"=w2972, "S4ACS_GUI in"=w2987) -> ("error out"=w2933:errorcluster, "S4ACS_GUI out"=w2934:refnum<class "S4GUI.lvclass">)  [unwired: 7 in]
        n1655 = call "Write cfg file.vi"("error in (no error)"=w2933, "cfg file"="lastsaved.cfg", "S4ACS_GUI in"=w2934) -> ("error out"=w2936:errorcluster, "S4ACS_GUI out"=w2937:refnum<class "S4GUI.lvclass">)  [unwired: 7 in]
      }
      event "Set from Input ch4": Value Change {
        n1656 = event-data() -> ()  [unwired: 1 in, 6 out]
        n1657 = local read "Input Cluster"() -> (w3012:T8)
        n1658 = Unbundle By Name(w3012) -> ("Parameters"=w3011:T5)
        n1659 = call-dynamic "Write User Event.vi"("error in (no error)"=w2991, "User Event"="SET CCD CONFIG CHANNEL4 ", "S4GUI in"=w2990) -> ("error out"=w2988:errorcluster, "S4GUI out"=w2989:refnum<class "S4GUI.lvclass">)  [unwired: 7 in]
        n1660 = Unbundle By Name(w3011) -> ("Image \nInitial Line"=w3039:u16, "Image\nInitial Column"=w3038:u16, "Image\nFinal Line"=w3037:u16, "Image\nFInal Column"=w3036:u16, "Vertical\nBinning"=w3035:u16, "Horizontal\nBinning"=w3034:u16, "Pre-amplification\nGain"=w3033:u8, "CCD\nEM Gain"=w3032:u16, "Readout\nRate"=w3031:u8, "Shutter\nOpenning Time"=w3030:i32, "Shutter\nClosing Time"=w3029:i32, "Vertical\nShift Speed"=w3028:u8, "Read\nMode"=w3027:u8, "Vertical\nClock Voltage"=w3026:u8, "A/D \nChannel"=w3025:u32, "Shutter\nMode"=w3024:u16, "Shutter\nTTL"=w3023:u16, "Trigger\nMode"=w3022:u16, "Frame\nTransfer"=w3002:bool, "Acquisition\nMode"=w3021:u8, "CCD \nEM Mode"=w3020:u8)
        n1661 = call-dynamic "Read AcquisitionD.vi"("error in (no error)"=w2988, "S4ACS_GUI in"=w2989) -> ("error out"=w3055:errorcluster, "Acquisition.lvclass"=w3058:refnum<class "Acquisition.lvclass">, "S4ACS_GUI out"=w3059:refnum<class "S4GUI.lvclass">)  [unwired: 7 in]
        n1662 = call-dynamic "Read Channel.vi"("error in (no error)"=w3055, "Acquisition in"=w3058) -> ("error out"=w3054:errorcluster, "Channel.lvclass"=w3056:refnum<class "Channel.lvclass">, "Acquisition out"=w3057:refnum<class "Acquisition.lvclass">)  [unwired: 7 in]
        n1663 = call-dynamic "Read Interface.vi"("error in (no error)"=w3054, "Channel in"=w3056) -> ("error out"=w3003:errorcluster, "Interface.lvclass"=w3004:refnum<class "Interface.lvclass">, "Channel out"=w2999:refnum<class "Channel.lvclass">)  [unwired: 7 in]
        n1664 = call-dynamic "Write PREV_FT.vi"("error in (no error)"=w3003, "PREV_FT"=w3002, "Interface in"=w3004) -> ("error out"=w2994:errorcluster, "Interface out"=w3000:refnum<class "Interface.lvclass">)  [unwired: 7 in]
        n1665 = call-dynamic "Read target cluster.vi"("error in (no error)"=w2994, "Channel in"=w2999) -> ("error out"=w3001:errorcluster, "target cluster"=w2998:T31, "Channel out"=w2997:refnum<class "Channel.lvclass">)  [unwired: 7 in]
        n1666 = Bundle By Name(cluster=w2998, "INITIAL_LINE"=w3039, "INITIAL_COLUMN"=w3038, "FINAL_LINE"=w3037, "FINAL_COLUMN"=w3036, "VBIN"=w3035, "HBIN"=w3034, "PREAMP"=w3033, "EM_GAIN"=w3032, "READOUT_RATE"=w3031, "SHUTTER_OPENING_TIME"=w3030, "SHUTTER_CLOSING_TIME"=w3029, "VERTICAL_SHIFT_SPEED"=w3028, "READ_MODE"=w3027, "VERTICAL_CLOCK_VOLTAGE"=w3026, "AD_CHANNEL"=w3025, "SHUTTER_MODE"=w3024, "SHUTTER_TTL"=w3023, "TRIGGER_MODE"=w3022, "FRAME_TRANSFER"=w3002, "ACQUISITION_MODE"=w3021, "EM_MODE"=w3020) -> (w2996:T31)
        n1667 = call-dynamic "Write target cluster.vi"("error in (no error)"=w3001, "target cluster"=w2996, "Channel in"=w2997) -> ("error out"=w2995:errorcluster, "Channel out"=w2993:refnum<class "Channel.lvclass">)  [unwired: 7 in]
        n1668 = Flatten To String(anything=w2996, error in (no error)=w2995) -> (data string=w3043:string, error out=w3042:errorcluster)  [unwired: 2 in, 1 out]
        n1669 = call "Write flatted cluster.vi"("error in (no error)"=w3042, "flatted cluster"=w3043, "Interface in"=w3000) -> ("error out"=w3041:errorcluster, "Interface out"=w3040:refnum<class "Interface.lvclass">)  [unwired: 7 in]
        n1670 = call-dynamic "Write Interface.vi"("error in (no error)"=w3041, "Interface.lvclass"=w3040, "Channel in"=w2993) -> ("error out"=w3015:errorcluster, "Channel out"=w3018:refnum<class "Channel.lvclass">)  [unwired: 7 in]
        n1671 = call "Write section_name.vi"("error in (no error)"=w3015, "section_name"="CCD_ACS4", "Channel in"=w3018) -> ("error out"=w3014:errorcluster, "Channel out"=w3017:refnum<class "Channel.lvclass">)  [unwired: 7 in]
        n1672 = call-dynamic "save config.vi"("error in (no error)"=w3014, "file config"="lastsaved.cfg", "Channel in"=w3017) -> ("error out"=w3013:errorcluster, "Channel out"=w3016:refnum<class "Channel.lvclass">)  [unwired: 7 in]
        n1673 = call-dynamic "Read State Machine.vi"("error in (no error)"=w3013, "Device in"=w3016) -> ("error out"=w3050:errorcluster, "State Machine.lvclass"=w3052:refnum<class "State Machine.lvclass">, "Device out"=w3053:refnum<class "Channel.lvclass">)  [unwired: 7 in]
        n1674 = call-dynamic "Write State.vi"("error in (no error)"=w3050, "State"=60, "State Machine in"=w3052) -> ("error out"=w3049:errorcluster, "State Machine out"=w3051:refnum<class "State Machine.lvclass">)  [unwired: 7 in]
        n1675 = call-dynamic "Write State Machine.vi"("error in (no error)"=w3049, "State Machine.lvclass"=w3051, "Device in"=w3053) -> ("error out"=w3046:errorcluster, "Device out"=w3047:refnum<class "Channel.lvclass">)  [unwired: 7 in]
        n1676 = call-dynamic "Write Channel.vi"("error in (no error)"=w3046, "Channel.lvclass"=w3047, "Acquisition in"=w3057) -> ("error out"=w3045:errorcluster, "Acquisition out"=w3044:refnum<class "Acquisition.lvclass">)  [unwired: 7 in]
        n1677 = call-dynamic "Write AcquisitionD.vi"("error in (no error)"=w3045, "Acquisition.lvclass"=w3044, "S4ACS_GUI in"=w3059) -> ("error out"=w3005:errorcluster, "S4ACS_GUI out"=w3006:refnum<class "S4GUI.lvclass">)  [unwired: 7 in]
        n1678 = call "Write cfg file.vi"("error in (no error)"=w3005, "cfg file"="lastsaved.cfg", "S4ACS_GUI in"=w3006) -> ("error out"=w3008:errorcluster, "S4ACS_GUI out"=w3009:refnum<class "S4GUI.lvclass">)  [unwired: 7 in]
      }
      event "Restore Default ch1": Value Change {
        n1679 = event-data() -> ()  [unwired: 1 in, 6 out]
        n1680 = call-dynamic "Read AcquisitionA.vi"("error in (no error)"=w3090, "S4ACS_GUI in"=w3091) -> ("error out"=w3086:errorcluster, "Acquisition.lvclass"=w3088:refnum<class "Acquisition.lvclass">, "S4ACS_GUI out"=w3089:refnum<class "S4GUI.lvclass">)  [unwired: 7 in]
        n1681 = call-dynamic "Read Channel.vi"("error in (no error)"=w3086, "Acquisition in"=w3088) -> ("error out"=w3073:errorcluster, "Channel.lvclass"=w3075:refnum<class "Channel.lvclass">, "Acquisition out"=w3087:refnum<class "Acquisition.lvclass">)  [unwired: 7 in]
        n1682 = call "Write section_name.vi"("error in (no error)"=w3073, "section_name"="CCD_ACS1", "Channel in"=w3075) -> ("error out"=w3072:errorcluster, "Channel out"=w3074:refnum<class "Channel.lvclass">)  [unwired: 7 in]
        n1683 = call-dynamic "load config.vi"("error in (no error)"=w3072, "cfg file name"="default.cfg", "Channel in"=w3074) -> ("error out"=w3070:errorcluster, "Channel out"=w3071:refnum<class "Channel.lvclass">)  [unwired: 7 in]
        n1684 = call-dynamic "Read State Machine.vi"("error in (no error)"=w3070, "Device in"=w3071) -> ("error out"=w3082:errorcluster, "State Machine.lvclass"=w3084:refnum<class "State Machine.lvclass">, "Device out"=w3085:refnum<class "Channel.lvclass">)  [unwired: 7 in]
        n1685 = call-dynamic "Write State.vi"("error in (no error)"=w3082, "State"=60, "State Machine in"=w3084) -> ("error out"=w3081:errorcluster, "State Machine out"=w3083:refnum<class "State Machine.lvclass">)  [unwired: 7 in]
        n1686 = call-dynamic "Write State Machine.vi"("error in (no error)"=w3081, "State Machine.lvclass"=w3083, "Device in"=w3085) -> ("error out"=w3066:errorcluster, "Device out"=w3062:refnum<class "Channel.lvclass">)  [unwired: 7 in]
        n1687 = call "Write section_name.vi"("error in (no error)"=w3066, "section_name"="CCD_ACS1", "Channel in"=w3062) -> ("error out"=w3067:errorcluster, "Channel out"=w3061:refnum<class "Channel.lvclass">)  [unwired: 7 in]
        n1688 = call-dynamic "save config.vi"("error in (no error)"=w3067, "file config"="lastsaved.cfg", "Channel in"=w3061) -> ("error out"=w3065:errorcluster, "Channel out"=w3060:refnum<class "Channel.lvclass">)  [unwired: 7 in]
        n1689 = call-dynamic "Write Channel.vi"("error in (no error)"=w3065, "Channel.lvclass"=w3060, "Acquisition in"=w3087) -> ("error out"=w3079:errorcluster, "Acquisition out"=w3078:refnum<class "Acquisition.lvclass">)  [unwired: 7 in]
        n1690 = call-dynamic "Write AcquisitionA.vi"("error in (no error)"=w3079, "Acquisition.lvclass"=w3078, "S4ACS_GUI in"=w3089) -> ("error out"=w3077:errorcluster, "S4ACS_GUI out"=w3068:refnum<class "S4GUI.lvclass">)  [unwired: 7 in]
      }
      event "Load Button": Value Change {
        (unwired) "C:\\Users\\observer\\sparc4\\s4gui\\Config" ("default name")
        n1691 = event-data() -> ()  [unwired: 1 in, 6 out]
        n1692 = String To Path(string="D:\\sparc4\\config\\s4gui" ("default name")) -> (path=w3095:path)
        n1693 = call "File Dialog"("start path"=w3095, "prompt"="Select file...", "button label"="Open", "default name"="lastsaved.cfg", "error in"=w3097, "pattern (all files)"="*.cfg") -> ("selected path"=w3094:path, "cancelled"=w3098:bool, "error out"=→"error out 2":errorcluster)  [unwired: 6 in, 1 out]
        n1694 = Strip Path(path=w3094) -> (name=w3093:string)  [unwired: 1 out]
        n1695 = case shown="False" w3098 {
          tunnel: w3105 -> [w3238 w3240]
          tunnel: [w3154 w3240] -> w3104
          tunnel: [w3152 w3239] -> w3103
          tunnel: w3097 -> [w3151 w3239]
          tunnel: w3093 -> [w3150 _]
          frame False {
            n1696 = call-dynamic "Read AcquisitionA.vi"("error in (no error)"=w3151, "S4ACS_GUI in"=w3238) -> ("error out"=w3234:errorcluster, "Acquisition.lvclass"=w3236:refnum<class "Acquisition.lvclass">, "S4ACS_GUI out"=w3237:refnum<class "S4GUI.lvclass">)  [unwired: 7 in]
            n1697 = call-dynamic "Read Channel.vi"("error in (no error)"=w3234, "Acquisition in"=w3236) -> ("error out"=w3221:errorcluster, "Channel.lvclass"=w3223:refnum<class "Channel.lvclass">, "Acquisition out"=w3235:refnum<class "Acquisition.lvclass">)  [unwired: 7 in]
            n1698 = call "Write section_name.vi"("error in (no error)"=w3221, "section_name"="CCD_ACS1", "Channel in"=w3223) -> ("error out"=w3220:errorcluster, "Channel out"=w3222:refnum<class "Channel.lvclass">)  [unwired: 7 in]
            n1699 = call-dynamic "load config.vi"("error in (no error)"=w3220, "cfg file name"=w3150, "Channel in"=w3222) -> ("error out"=w3148:errorcluster, "Channel out"=w3149:refnum<class "Channel.lvclass">)  [unwired: 7 in]
            n1700 = call-dynamic "save config.vi"("error in (no error)"=w3148, "file config"="lastsaved.cfg", "Channel in"=w3149) -> ("error out"=w3130:errorcluster, "Channel out"=w3131:refnum<class "Channel.lvclass">)  [unwired: 7 in]
            n1701 = call-dynamic "Read target cluster.vi"("error in (no error)"=w3130, "Channel in"=w3131) -> ("target cluster"=w3106:T31)  [unwired: 7 in, 2 out]
            n1702 = call-dynamic "Read State Machine.vi"("error in (no error)"=w3130, "Device in"=w3131) -> ("error out"=w3230:errorcluster, "State Machine.lvclass"=w3232:refnum<class "State Machine.lvclass">, "Device out"=w3233:refnum<class "Channel.lvclass">)  [unwired: 7 in]
            n1703 = call-dynamic "Write State.vi"("error in (no error)"=w3230, "State"=60, "State Machine in"=w3232) -> ("error out"=w3229:errorcluster, "State Machine out"=w3231:refnum<class "State Machine.lvclass">)  [unwired: 7 in]
            n1704 = call-dynamic "Write State Machine.vi"("error in (no error)"=w3229, "State Machine.lvclass"=w3231, "Device in"=w3233) -> ("error out"=w3226:errorcluster, "Device out"=w3227:refnum<class "Channel.lvclass">)  [unwired: 7 in]
            n1705 = call-dynamic "Write Channel.vi"("error in (no error)"=w3226, "Channel.lvclass"=w3227, "Acquisition in"=w3235) -> ("error out"=w3225:errorcluster, "Acquisition out"=w3224:refnum<class "Acquisition.lvclass">)  [unwired: 7 in]
            n1706 = call-dynamic "Write AcquisitionA.vi"("error in (no error)"=w3225, "Acquisition.lvclass"=w3224, "S4ACS_GUI in"=w3237) -> ("error out"=w3161:errorcluster, "S4ACS_GUI out"=w3160:refnum<class "S4GUI.lvclass">)  [unwired: 7 in]
            n1707 = call "Read AcquisitionB.vi"("error in (no error)"=w3161, "S4ACS_GUI in"=w3160) -> ("error out"=w3203:errorcluster, "Acquisition.lvclass"=w3201:refnum<class "Acquisition.lvclass">, "S4ACS_GUI out"=w3200:refnum<class "S4GUI.lvclass">)  [unwired: 7 in]
            n1708 = call-dynamic "Read Channel.vi"("error in (no error)"=w3203, "Acquisition in"=w3201) -> ("error out"=w3216:errorcluster, "Channel.lvclass"=w3214:refnum<class "Channel.lvclass">, "Acquisition out"=w3202:refnum<class "Acquisition.lvclass">)  [unwired: 7 in]
            n1709 = call "Write section_name.vi"("error in (no error)"=w3216, "section_name"="CCD_ACS2", "Channel in"=w3214) -> ("error out"=w3217:errorcluster, "Channel out"=w3215:refnum<class "Channel.lvclass">)  [unwired: 7 in]
            n1710 = call-dynamic "load config.vi"("error in (no error)"=w3217, "cfg file name"=w3150, "Channel in"=w3215) -> ("error out"=w3145:errorcluster, "Channel out"=w3143:refnum<class "Channel.lvclass">)  [unwired: 7 in]
            n1711 = call-dynamic "save config.vi"("error in (no error)"=w3145, "file config"="lastsaved.cfg", "Channel in"=w3143) -> ("error out"=w3144:errorcluster, "Channel out"=w3142:refnum<class "Channel.lvclass">)  [unwired: 7 in]
            n1712 = call-dynamic "Read State Machine.vi"("error in (no error)"=w3144, "Device in"=w3142) -> ("error out"=w3207:errorcluster, "State Machine.lvclass"=w3205:refnum<class "State Machine.lvclass">, "Device out"=w3204:refnum<class "Channel.lvclass">)  [unwired: 7 in]
            n1713 = call-dynamic "Write State.vi"("error in (no error)"=w3207, "State"=60, "State Machine in"=w3205) -> ("error out"=w3208:errorcluster, "State Machine out"=w3206:refnum<class "State Machine.lvclass">)  [unwired: 7 in]
            n1714 = call-dynamic "Write State Machine.vi"("error in (no error)"=w3208, "State Machine.lvclass"=w3206, "Device in"=w3204) -> ("error out"=w3211:errorcluster, "Device out"=w3210:refnum<class "Channel.lvclass">)  [unwired: 7 in]
            n1715 = call-dynamic "Write Channel.vi"("error in (no error)"=w3211, "Channel.lvclass"=w3210, "Acquisition in"=w3202) -> ("error out"=w3212:errorcluster, "Acquisition out"=w3213:refnum<class "Acquisition.lvclass">)  [unwired: 7 in]
            n1716 = call "Write AcquisitionB.vi"("error in (no error)"=w3212, "Acquisition.lvclass"=w3213, "S4ACS_GUI in"=w3200) -> ("error out"=w3159:errorcluster, "S4ACS_GUI out"=w3158:refnum<class "S4GUI.lvclass">)  [unwired: 7 in]
            n1717 = call-dynamic "Read AcquisitionC.vi"("error in (no error)"=w3159, "S4ACS_GUI in"=w3158) -> ("error out"=w3196:errorcluster, "Acquisition.lvclass"=w3198:refnum<class "Acquisition.lvclass">, "S4ACS_GUI out"=w3199:refnum<class "S4GUI.lvclass">)  [unwired: 7 in]
            n1718 = call-dynamic "Read Channel.vi"("error in (no error)"=w3196, "Acquisition in"=w3198) -> ("error out"=w3183:errorcluster, "Channel.lvclass"=w3185:refnum<class "Channel.lvclass">, "Acquisition out"=w3197:refnum<class "Acquisition.lvclass">)  [unwired: 7 in]
            n1719 = call "Write section_name.vi"("error in (no error)"=w3183, "section_name"="CCD_ACS3", "Channel in"=w3185) -> ("error out"=w3182:errorcluster, "Channel out"=w3184:refnum<class "Channel.lvclass">)  [unwired: 7 in]
            n1720 = call-dynamic "load config.vi"("error in (no error)"=w3182, "cfg file name"=w3150, "Channel in"=w3184) -> ("error out"=w3140:errorcluster, "Channel out"=w3138:refnum<class "Channel.lvclass">)  [unwired: 7 in]
            n1721 = call-dynamic "save config.vi"("error in (no error)"=w3140, "file config"="lastsaved.cfg", "Channel in"=w3138) -> ("error out"=w3139:errorcluster, "Channel out"=w3137:refnum<class "Channel.lvclass">)  [unwired: 7 in]
            n1722 = call-dynamic "Read State Machine.vi"("error in (no error)"=w3139, "Device in"=w3137) -> ("error out"=w3192:errorcluster, "State Machine.lvclass"=w3194:refnum<class "State Machine.lvclass">, "Device out"=w3195:refnum<class "Channel.lvclass">)  [unwired: 7 in]
            n1723 = call-dynamic "Write State.vi"("error in (no error)"=w3192, "State"=60, "State Machine in"=w3194) -> ("error out"=w3191:errorcluster, "State Machine out"=w3193:refnum<class "State Machine.lvclass">)  [unwired: 7 in]
